vi "Configure Output Protection.vi"(0 "VISA resource name":refnum<visa-resource-name>, 5 "Voltage Limit (0 volts)":dbl, 7 "Current Limit (0 amperes)":dbl, 9 "Power Limit (0 watts)":dbl, 11 "error in (no error)":errorcluster) -> (4 "VISA resource name out":refnum<visa-resource-name>, 15 "error out":errorcluster)   [LabVIEW 2018, in "XP Power PLS600.lvlib"]
doc: "Configures the over-voltage protection (OVP) threshold in volts, over-current protection (OCP) threshold in amperes, and over-power protection (OPP) threshold in watts."
uses:
  XP Power PLS600.lvlib
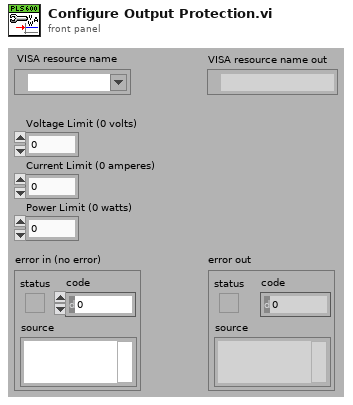
[diagram p1: front panel]
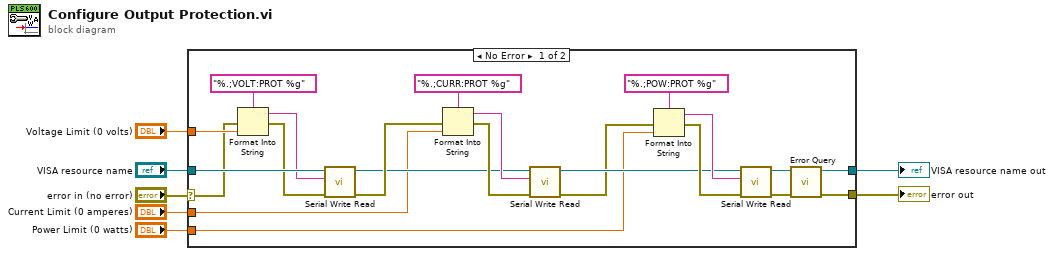
[diagram p0: block diagram]
diagram:
  n1 = case shown="No Error" "error in (no error)" {
    selector: "error in (no error)" -> [w24 w30]
    tunnel: "Voltage Limit (0 volts)" -> [w28 _]
    tunnel: [w11 w31] -> w6
    tunnel: [w12 w30] -> w5
    tunnel: "VISA resource name" -> [w27 w31]
    tunnel: "Current Limit (0 amperes)" -> [w10 _]
    tunnel: "Power Limit (0 watts)" -> [w9 _]
    frame No Error {
      n2 = Format Into String(format string="%.;VOLT:PROT %g", error in=w24, w28) -> (resulting string=w26:string, error out=w25:errorcluster)  [unwired: 1 in]
      n3 = call "Serial Write Read.vi"("error in (no error)"=w25, "Write Buffer"=w26, "VISA resource name"=w27) -> ("error out"=w15:errorcluster, "VISA resource name out"=w14:refnum<visa-resource-name>)  [unwired: 6 in, 1 out]
      n4 = Format Into String(format string="%.;CURR:PROT %g", error in=w15, w10) -> (resulting string=w22:string, error out=w21:errorcluster)  [unwired: 1 in]
      n5 = call "Serial Write Read.vi"("error in (no error)"=w21, "Write Buffer"=w22, "VISA resource name"=w14) -> ("error out"=w8:errorcluster, "VISA resource name out"=w13:refnum<visa-resource-name>)  [unwired: 6 in, 1 out]
      n6 = Format Into String(format string="%.;POW:PROT %g", error in=w8, w9) -> (resulting string=w19:string, error out=w18:errorcluster)  [unwired: 1 in]
      n7 = call "Serial Write Read.vi"("error in (no error)"=w18, "Write Buffer"=w19, "VISA resource name"=w13) -> ("error out"=w16:errorcluster, "VISA resource name out"=w17:refnum<visa-resource-name>)  [unwired: 6 in, 1 out]
      n8 = call "Error Query.vi"("error in (no error)"=w16, "VISA resource name"=w17) -> ("error out"=w12:errorcluster, "VISA resource name out"=w11:refnum<visa-resource-name>)  [unwired: 6 in, 2 out]
    }
    frame Error {
    }
  }
  "VISA resource name out" <- w6
  "error out" <- w5
